vi "Testing Flag (library variable).vi"() -> ()   [LabVIEW 2021]
uses:
  Testing Flag (enum).ctl
panel:
  in  "Testing Flag":T1
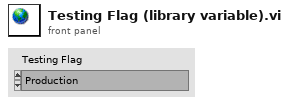
[diagram p1: front panel]
types:
  T1 = typedef "Testing Flag (enum).ctl" = enum16{"Production", "Testing"}
diagram:
